vi "P1_MechanicalActions.vi"() -> ()   [LabVIEW 2022 SP3]
panel:
  out "SWP 6":bool
  out "SWP 5":bool
  out "SWP 4":bool
  out "SWP 3":bool
  out "SWP 2":bool
  in  "Latch until released":bool
  in  "Latch when released":bool
  in  "Latch when pressed":bool
  in  "Switch until released":bool
  in  "Switch when released":bool
  in  "?":bool
  out "SWP":bool
  in  "Switch when pressed":bool
  # "MECHANICAL ACTIONS"
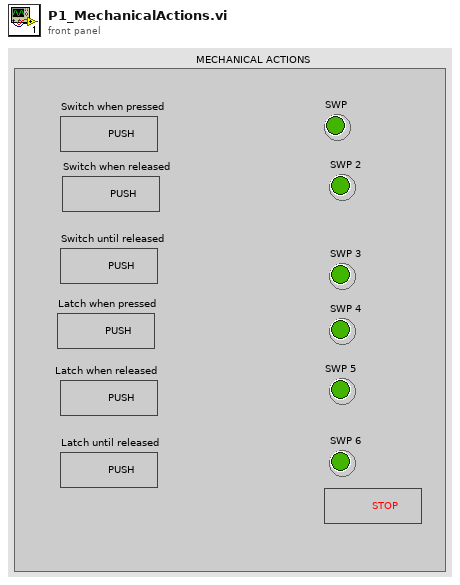
[diagram p1: front panel]
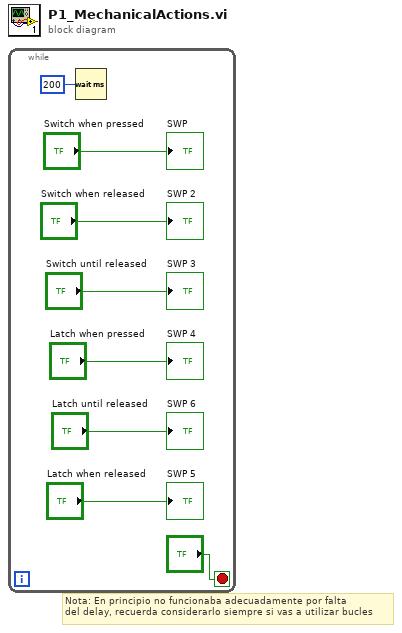
[diagram p0: block diagram]
diagram:
  # "Nota: En principio no funcionaba adecuadamente por falta\ndel delay, recuerda considerarlo siempre si vas a utilizar bucles"
  n1 = while {
    stop <- "?" stop-if-true
    n2 = Wait (ms)(milliseconds to wait=u32 200 ("millisecond timer value")) -> ()  [unwired: 1 out]
    "SWP" <- "Switch when pressed"
    "SWP 2" <- "Switch when released"
    "SWP 3" <- "Switch until released"
    "SWP 4" <- "Latch when pressed"
    "SWP 5" <- "Latch when released"
    "SWP 6" <- "Latch until released"
  }
